vi "configDotNetMember(arrayParam).vi"(0 "dotNetModule":refnum<k7>, 5 "Index array":i32[](array[numeric]), 7 "Parameter Value array":string[][](array[string]), 11 "error in (no error)":errorcluster) -> (15 "error out":errorcluster)   [LabVIEW 2010]
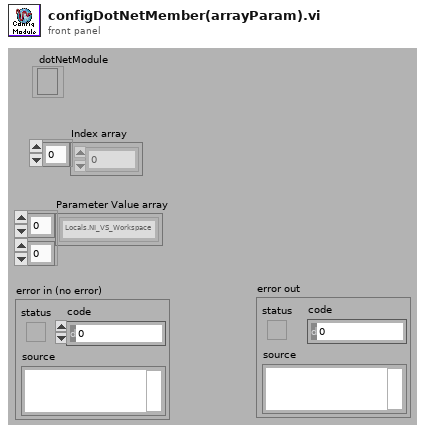
[diagram p1: front panel]
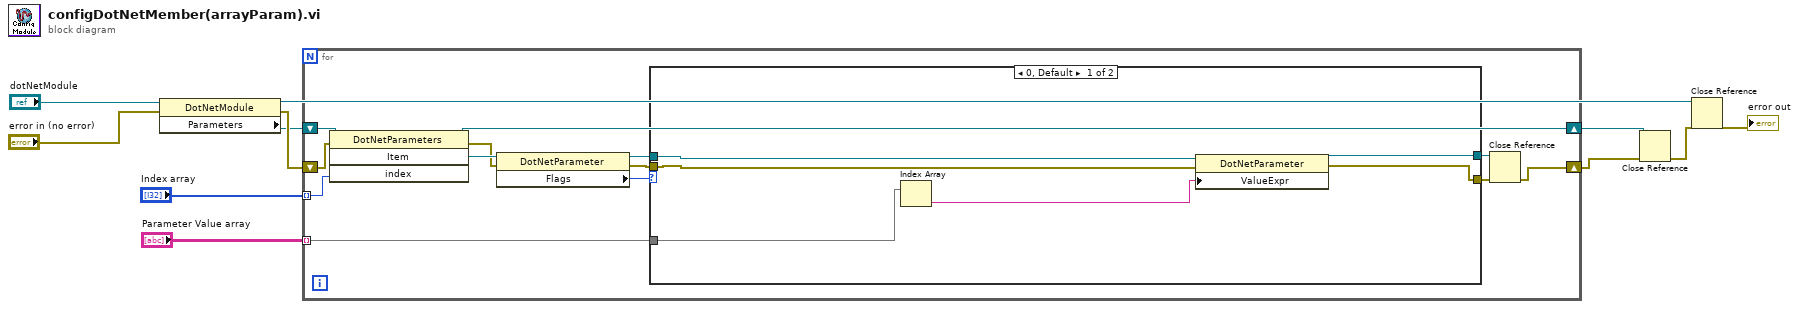
[diagram p0: block diagram]
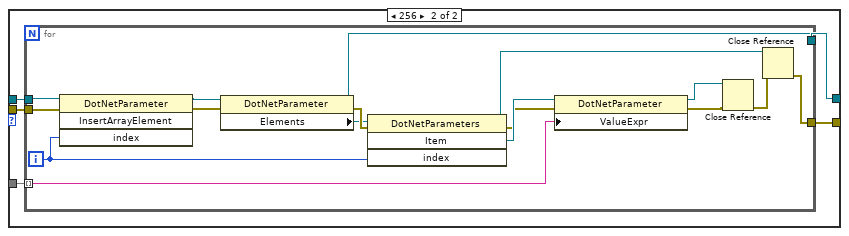
[diagram p2: hidden frame]
diagram:
  n1 = property class="DotNetModule"(reference="dotNetModule", error in="error in (no error)") -> (reference out=w4:refnum<k7>, error out=w11:errorcluster, "Parameters"=w8:refnum<k7>)
  n2 = for {
    tunnel: "Index array" -> [w22] mode=indexing
    tunnel: "Parameter Value array" -> [w21] mode=indexing
    shift-right: [w18] -> w1
    shift-left: w11 -> [w24]
    shift-right: [w23] -> w9
    shift-left: w8 -> [w12]
    n3 = invoke class="DotNetParameters" method="Item"(reference=w12, error in=w24, "index"=w22) -> (reference out=w23:refnum<k7>, error out=w16:errorcluster, "Item"=w17:refnum<k7>)  [unwired: 1 in, 1 out]
    n4 = property class="DotNetParameter"(reference=w17, error in=w16) -> (reference out=w14:refnum<k7>, error out=w13:errorcluster, "Flags"=w15:i32)
    n5 = case shown="0, Default" w15 {
      tunnel: w21 -> [w26 w35]
      tunnel: [w30 w33] -> w20
      tunnel: [w29 w34] -> w19
      tunnel: w14 -> [w28 w32]
      tunnel: w13 -> [w27 w31]
      frame 0, Default {
        n6 = Index Array(array=w26) -> (element=w25:string)  [unwired: 1 in]
        n7 = property class="DotNetParameter"(reference=w28, error in=w27, "ValueExpr"=w25) -> (reference out=w30:refnum<k7>, error out=w29:errorcluster)
      }
      frame 256 {
        n8 = for {
          tunnel: w35 -> [w51] mode=indexing
          tunnel: [w43] -> w34
          tunnel: [w42] -> w33
          tunnel: w32 -> [w40]
          tunnel: w31 -> [w37]
          i -> [w36]
          n9 = invoke class="DotNetParameter" method="InsertArrayElement"(reference=w40, error in=w37, "index"=w36) -> (reference out=w41:refnum<k7>, error out=w39:errorcluster)  [unwired: 1 in, 2 out]
          n10 = property class="DotNetParameter"(reference=w41, error in=w39) -> (reference out=w42:refnum<k7>, error out=w48:errorcluster, "Elements"=w47:refnum<k7>)
          n11 = invoke class="DotNetParameters" method="Item"(reference=w47, error in=w48, "index"=w36) -> (reference out=w44:refnum<k7>, error out=w38:errorcluster, "Item"=w50:refnum<k7>)  [unwired: 1 in, 1 out]
          n12 = property class="DotNetParameter"(reference=w50, error in=w38, "ValueExpr"=w51) -> (reference out=w46:refnum<k7>, error out=w49:errorcluster)
          n13 = Close Reference(reference=w46, error in (no error)=w49) -> (error out=w45:errorcluster)
          n14 = Close Reference(reference=w44, error in (no error)=w45) -> (error out=w43:errorcluster)
        }
      }
    }
    n15 = Close Reference(reference=w20, error in (no error)=w19) -> (error out=w18:errorcluster)
  }
  n16 = Close Reference(reference=w9, error in (no error)=w1) -> (error out=w3:errorcluster)
  n17 = Close Reference(reference=w4, error in (no error)=w3) -> (error out=→"error out":errorcluster)
